vi "Robot Main.vi"() -> ()   [LabVIEW 2013]
doc: "This VI imlements the framework and scheduler for your robotics program. It should not be necessary to modify the framework. You are expected to add your code to the VIs called from Robot Main, the ones located in the Team Code within the project."
uses:
  Robot Global Data.vi
panel:
  in  "Finish":bool
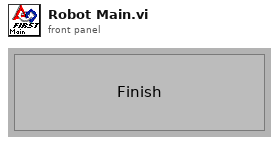
[diagram p1: front panel]
types:
  T1 = typedef "WPI_DriverStationMatch Info.ctl" = cluster{"Autonomous Elapsed Seconds":dbl, "TeleOp Elapsed Seconds":dbl, "Disabled Elapsed Seconds":dbl, "Visited Autonomous":bool, "Visited TeleOp":bool, "Visited Disabled":bool, "Autonomous Settings":cluster{"Autonomous Style":enum16{"Iterative", "Independent"}, "VI Refnum":refnum<vi>}}
  T2 = typedef "WPI_DriverStationDerivedRobotMode.ctl" = enum16{"Init", "Execute", "Stop"}
  T3 = typedef "WPI_DriverStationRobotMode2.ctl" = enum16{"Autonomous Disabled", "Autonomous Enabled", "Teleop Disabled", "Teleop Enabled", "Timeout", "Finish", "Test Disabled", "Test Enabled"}
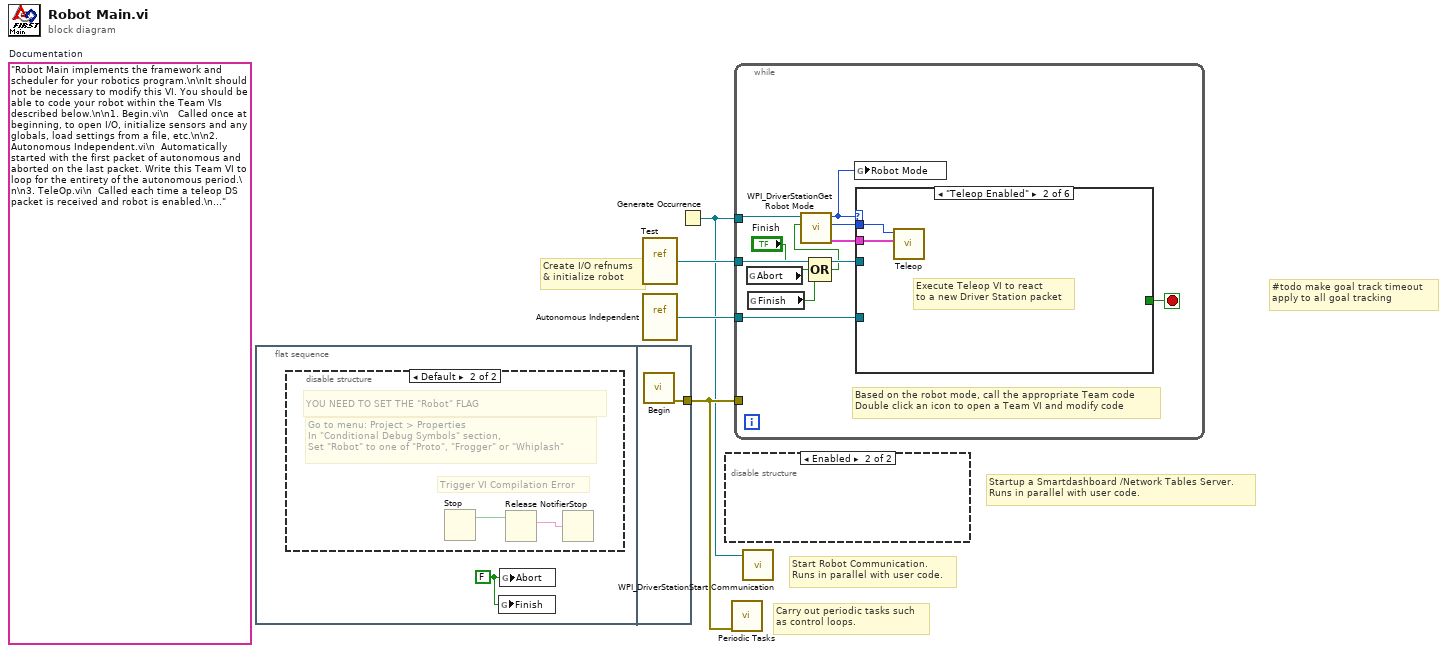
[diagram p0: block diagram]
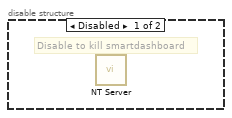
[diagram p2: hidden frame]
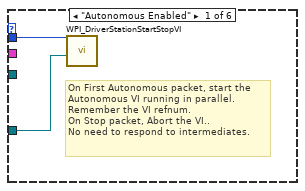
[diagram p4: hidden frame]
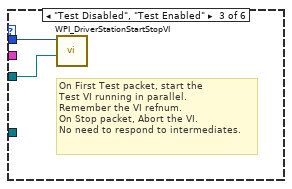
[diagram p5: hidden frame]
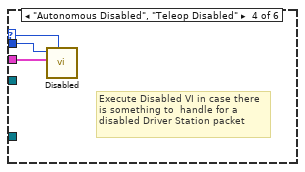
[diagram p6: hidden frame]
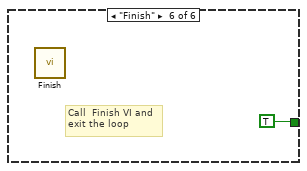
[diagram p8: hidden frame]
diagram:
  (unwired) "Robot Main implements the framework and scheduler for your robotics program.\n\nIt should not be necessary to modify this VI. You should be able to code your robot within the Team VIs described below.\n\n1. Begin.vi\n   Called once at beginning, to open I/O, initialize sensors and any globals, load settings from a file, etc.\n\n2. Autonomous Independent.vi\n  Automatically started with the first packet of autonomous and aborted on the last packet. Write this Team VI to loop for the entirety of the autonomous period.\n\n3. TeleOp.vi\n  Called each time a teleop DS packet is received and robot is enabled.\n\n4. Disabled.vi\n  Called each time a packet is received and the robot is disabled.\n\n5. Test.vi\n  Called Automatically started with the first test packet and aborted on the last. Modify this VI to carry out robot and sensor validation tests.\n\n6. Vision.vi\n  A parallel loop that acquires and processes camera images.\n\n7. PeriodicTasks.vi\n  Parallel loops running at user-defined rates.\n\n8. Finish.vi\n  Called before exiting, so you can save data, clean up I/O, etc.\n"  # Documentation
  # "#todo make goal track timeout\napply to all goal tracking"
  # "Startup a Smartdashboard /Network Tables Server.\nRuns in parallel with user code."
  # "Carry out periodic tasks such\nas control loops."
  # "Create I/O refnums\n& initialize robot"
  # "Start Robot Communication.\nRuns in parallel with user code."
  n1 = flat-sequence {
    tunnel: [w8] -> w2
    frame #0 {
      w5 = FALSE ("Abort")
      n2 = disable-structure shown="Default" {
        frame condition #0 (active) {
        }
        frame condition #1 {
          # "Go to menu: Project > Properties\nIn \"Conditional Debug Symbols\" section,\nSet \"Robot\" to one of \"Proto\", \"Frogger\" or \"Whiplash\""
          # "YOU NEED TO SET THE \"Robot\" FLAG"
          # "Trigger VI Compilation Error"
          n3 = Stop() -> (stop? (T)=w7:bool)
          n4 = Release Notifier(notifier=w7) -> (last notification=w6:string)  [unwired: 2 in, 2 out]
          n5 = Stop(stop? (T)=w6) -> ()
        }
      }
      n6 = global write "Robot Global Data.vi" "Finish"(w5) -> ()
      n7 = global write "Robot Global Data.vi" "Abort"(w5) -> ()
    }
    frame #1 {
      n8 = call "Begin.vi"() -> ("error out"=w8:errorcluster)  [unwired: 1 in, 10 out]
    }
  }
  n9 = vi-ref "Test.vi"() -> (w3:refnum<vi>)
  n10 = vi-ref "Autonomous Independent.vi"() -> (w4:refnum<vi>)
  n11 = Generate Occurrence() -> (w1:refnum<k4>)
  n12 = disable-structure shown="Enabled" {
    frame Disabled {
      # "Disable to kill smartdashboard"
      n13 = call <vilib>:"NT Server.vi"() -> ()  [unwired: 12 in]
    }
    frame Enabled {
    }
  }
  n14 = call "Periodic Tasks.vi"("error in"=w2) -> ()  [unwired: 2 in, 9 out]
  n15 = while "Scheduling loop" {
    tunnel: w1 -> [w18]
    tunnel: w4 -> [w15]
    tunnel: w3 -> [w14]
    tunnel: w2 -> [_]
    stop <- w16 stop-if-true
    # "Based on the robot mode, call the appropriate Team code\nDouble click an icon to open a Team VI and modify code"
    n16 = global read "Robot Global Data.vi" "Abort"() -> (w11:bool)
    n17 = global read "Robot Global Data.vi" "Finish"() -> (w12:bool)
    n18 = Compound Arithmetic op=OR("Finish", w11, w12) -> (w9:bool)
    n19 = call <vilib>:"WPI_DriverStationGet Robot Mode.vi"("Finish"=w9, "DS Occurrence"=w18) -> ("Match Info out"=w17:T1, "Call Context"=w19:T2, "Robot Mode"=w13:T3)  [unwired: 7 out]
    n20 = global write "Robot Global Data.vi" "Robot Mode"(w13) -> ()
    n21 = case shown="\"Teleop Enabled\"" w13 {
      selector: w13 -> [_ _ _ w26 _ _]
      tunnel: w19 -> [w21 w23 w25 w28 _ _]
      tunnel: w17 -> [_ w22 _ w27 _ _]
      tunnel: [_ _ _ _ _ TRUE] -> w16
      tunnel: w15 -> [w20 _ _ _ _ _]
      tunnel: w14 -> [_ _ w24 _ _ _]
      frame "Autonomous Enabled" {
        # "On First Autonomous packet, start the\nAutonomous VI running in parallel.\nRemember the VI refnum.\nOn Stop packet, Abort the VI..\nNo need to respond to intermediates."
        n22 = call <vilib>:"WPI_DriverStationStartStopVI.vi"("VI in"=w20, "Call Context"=w21) -> ()  [unwired: 10 in]
      }
      frame "Teleop Enabled" {
        # "Execute Teleop VI to react\nto a new Driver Station packet"
        n23 = call "Teleop.vi"("Match Info"=w22, "Call Context"=w23) -> ()  [unwired: 1 in, 9 out]
      }
      frame "Test Disabled", "Test Enabled" {
        # "On First Test packet, start the\nTest VI running in parallel.\nRemember the VI refnum.\nOn Stop packet, Abort the VI.\nNo need to respond to intermediates."
        n24 = call <vilib>:"WPI_DriverStationStartStopVI.vi"("VI in"=w24, "Call Context"=w25) -> ()  [unwired: 10 in]
      }
      frame "Autonomous Disabled", "Teleop Disabled" {
        # "Execute Disabled VI in case there\nis something to  handle for a\ndisabled Driver Station packet"
        n25 = call "Disabled.vi"("Robot Mode"=w26, "Match Info"=w27, "Call Context"=w28) -> ()  [unwired: 1 in, 8 out]
      }
      frame "Timeout" {
        # "Driver Station packet didn't arrive.\nPossibly useful for diagnostics"
      }
      frame "Finish" {
        # "Call  Finish VI and\nexit the loop"
        n26 = call "Finish.vi"() -> ()  [unwired: 1 in, 7 out]
      }
    }
  }
  n27 = call <vilib>:"WPI_DriverStationStart Communication.vi"("occurrence"=w1) -> ()  [unwired: 11 in]
